vi "Read controller temp test.vi"() -> ()   [LabVIEW 2023]
panel:
  out "error out 2":errorcluster
  in  "stop 2":bool
  in  "VISA Refnum in":refnum<visa-resource-name>
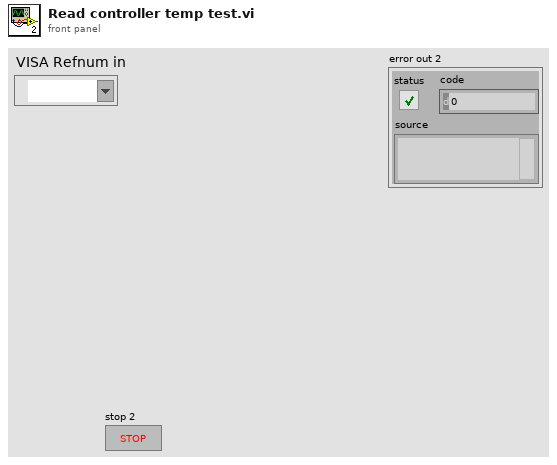
[diagram p1: front panel]
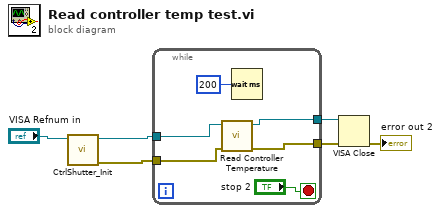
[diagram p0: block diagram]
diagram:
  n1 = call "CtrlShutter_Init.vi"("VISA Refnum in"="VISA Refnum in") -> ("error out"=w2:errorcluster, "VISA Refnum out"=w1:refnum<visa-resource-name>)  [unwired: 8 in, 1 out]
  n2 = while {
    tunnel: w1 -> [w7]
    tunnel: w2 -> [w8]
    tunnel: [w10] -> w6
    tunnel: [w9] -> w5
    stop <- "stop 2" stop-if-true
    n3 = call "Read Controller Temperature.vi"("VISA Refnum in"=w7, "error in (no error)"=w8) -> ("VISA Refnum out"=w10:refnum<visa-resource-name>, "error out"=w9:errorcluster)  [unwired: 6 in, 1 out]
    n4 = Wait (ms)(milliseconds to wait=u32 200) -> ()  [unwired: 1 out]
  }
  n5 = VISA Close(VISA resource name=w6, error in (no error)=w5) -> (error out=→"error out 2":errorcluster)
